vi "DisplayProperties.vi"(11 "Class In":refnum<class "SamplerPluginsBase.lvclass">) -> (3 "Class out":refnum<class "SamplerPluginsBase.lvclass">)   [LabVIEW 2014, in "SamplerPlugins.lvlib" / "SamplerPluginsBase.lvclass"]
uses:
  SamplerPluginsBase.lvclass
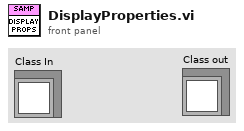
[diagram p1: front panel]
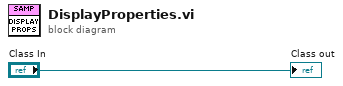
[diagram p0: block diagram]
diagram:
  "Class out" <- "Class In"
